vi "GetRefDatafromINIFile.vi"(8 "error in (no error)":errorcluster, 11 "RefDataIn":string) -> (0 "error out":errorcluster, 2 "DNUMList":i32[](array[numeric]), 3 "Reference Data":dbl[][](array[numeric]))   [LabVIEW 2019]
uses:
  <vilib>/Utility/config.llb/Read Key (Double).vi
  <vilib>/Utility/config.llb/NI_LVConfig.lvlib
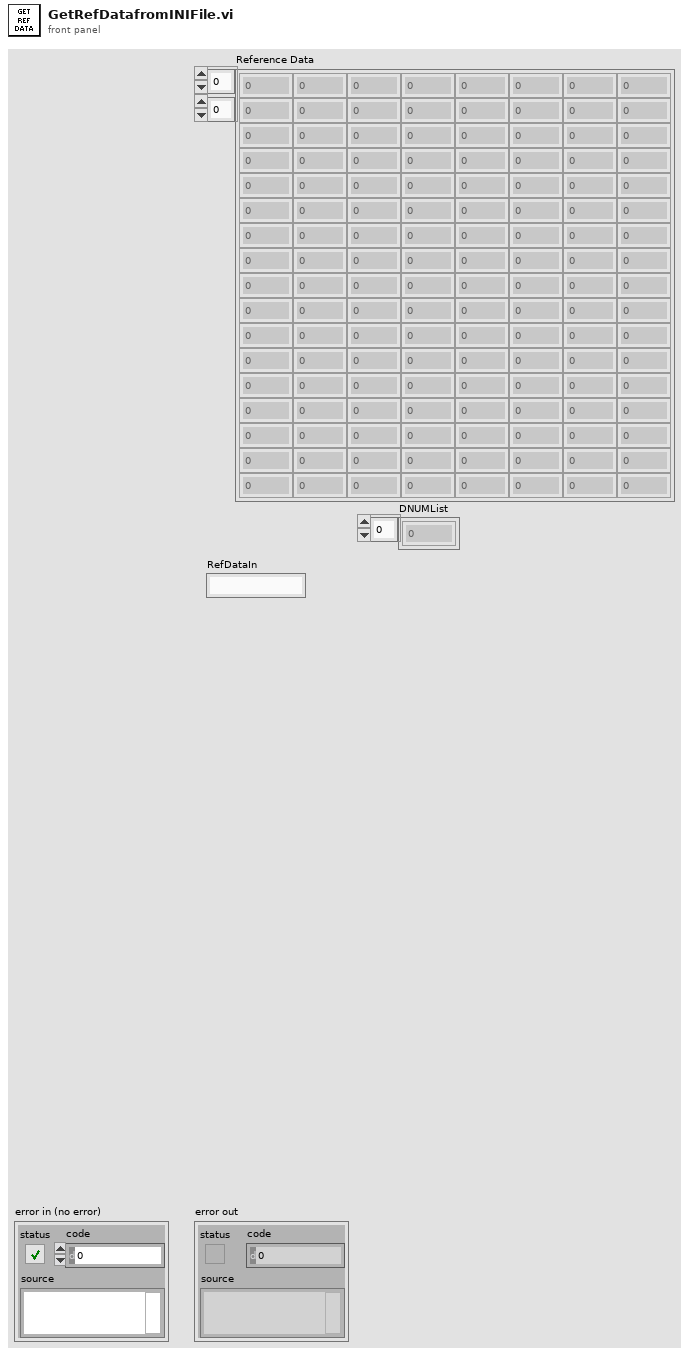
[diagram p1: front panel]
types:
  T1 = typedef "NI_LVConfig.lvlib/Config Data RefNum.ctl" = refnum<k1>
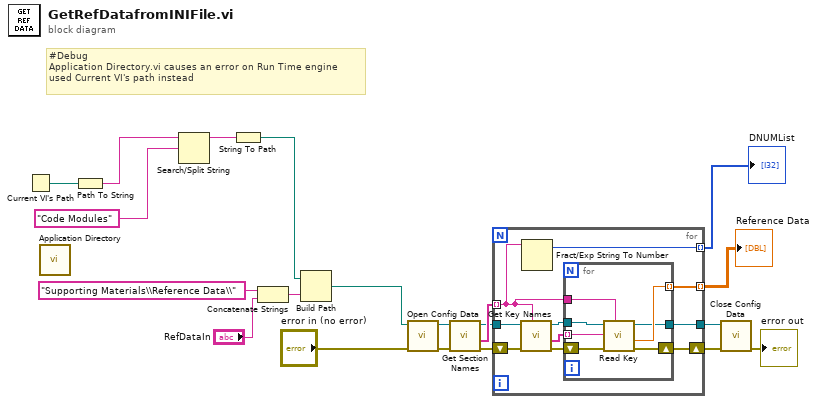
[diagram p0: block diagram]
diagram:
  # "#Debug\nApplication Directory.vi causes an error on Run Time engine\nused Current VI's path instead"
  n1 = Current VI's Path() -> (path=w5:path)
  n2 = call <vilib>:"Application Directory.vi"() -> ()  [unwired: 1 out]
  n3 = Path To String(path=w5) -> (string=w4:string)
  n4 = Search/Split String(string=w4, search string/char (-)="Code Modules") -> (substring before match=w2:string)  [unwired: 1 in, 2 out]
  n5 = String To Path(string=w2) -> (path=w1:path)
  n6 = Concatenate Strings("Supporting Materials\\Reference Data\\" ("name or relative path"), "RefDataIn") -> (w8:string)
  n7 = Build Path(base path=w1, name or relative path=w8) -> (appended path=w6:path)
  n8 = call <vilib>:"Open Config Data.vi"("error in (no error)"="error in (no error)", "configuration file path"=w6) -> ("error out"=w16:errorcluster, "refnum"=w20:T1)  [unwired: 7 in, 1 out]
  n9 = call <vilib>:"Get Section Names.vi"("error in (no error)"=w16, "refnum"=w20) -> ("error out"=w15:errorcluster, "section names"=w19:string[], "refnum out"=w18:T1)  [unwired: 7 in]
  n10 = for {
    tunnel: w19 -> [w22] mode=indexing
    tunnel: w18 -> [w30]
    tunnel: [w27] -> w17 mode=indexing
    shift-right: [w24] -> w12
    shift-left: w15 -> [w26]
    tunnel: [w23] -> w13
    tunnel: [w21] -> w10 mode=indexing
    n11 = call <vilib>:"Get Key Names.vi"("section"=w22, "error in (no error)"=w26, "refnum"=w30) -> ("error out"=w25:errorcluster, "key names"=w29:string[], "refnum out"=w28:T1)  [unwired: 5 in, 1 out]
    n12 = Fract/Exp String To Number(string=w22) -> (offset past number=w21:i32)  [unwired: 3 in, 1 out]
    n13 = for {
      tunnel: w29 -> [w36] mode=indexing
      tunnel: w28 -> [w37]
      tunnel: w22 -> [w35]
      tunnel: [w34] -> w27 mode=indexing
      shift-right: [w32] -> w24
      shift-left: w25 -> [w33]
      tunnel: [w31] -> w23
      n14 = call-poly <vilib>:"Read Key.vi"("section"=w35, "error in (no error)"=w33, "key"=w36, "refnum"=w37) -> ("error out"=w32:errorcluster, "value"=w34:dbl, "refnum out"=w31:T1)  [unwired: 4 in, 1 out]
    }
  }
  "Reference Data" <- w17
  "DNUMList" <- w10
  n15 = call <vilib>:"Close Config Data.vi"("error in (no error)"=w12, "refnum"=w13) -> ("error out"=→"error out":errorcluster)  [unwired: 8 in, 1 out]
